vi "Extract Project Strings.vi"(8 "error in (no error)":errorcluster, 11 "New Project Wizard in":refnum<class "New Project Wizard.lvclass">) -> (0 "error out":errorcluster, 3 "New Project Wizard out":refnum<class "New Project Wizard.lvclass">)   [LabVIEW 2013, in "SET Project Editor.lvlib" / "New Project Wizard.lvclass"]
uses:
  New Project Wizard.lvclass
  New Project Wizard.lvclass/New Project Wizard.ctl
  SET Project Data/Resource Data Class/Resource Data.lvclass
  SET Project Data/Project Data Class/Project Data.lvclass
  SET Project Data/VI Class/VI Data.lvclass
  SET Project Data/Menu Class/Menu Data.lvclass
  lib/printf/messages/General/LV_Printf Msg.lvclass
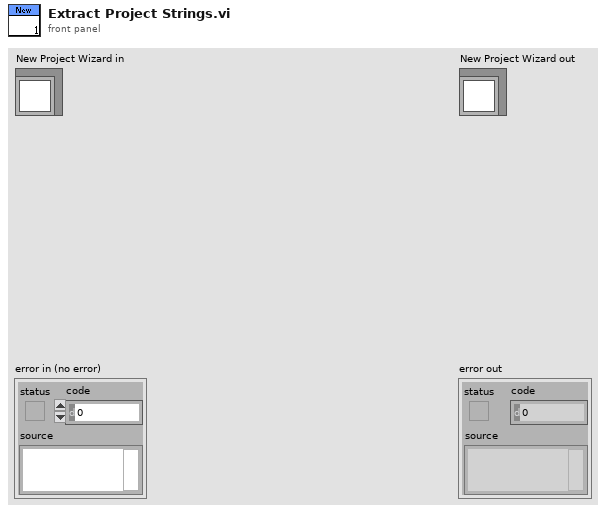
[diagram p1: front panel]
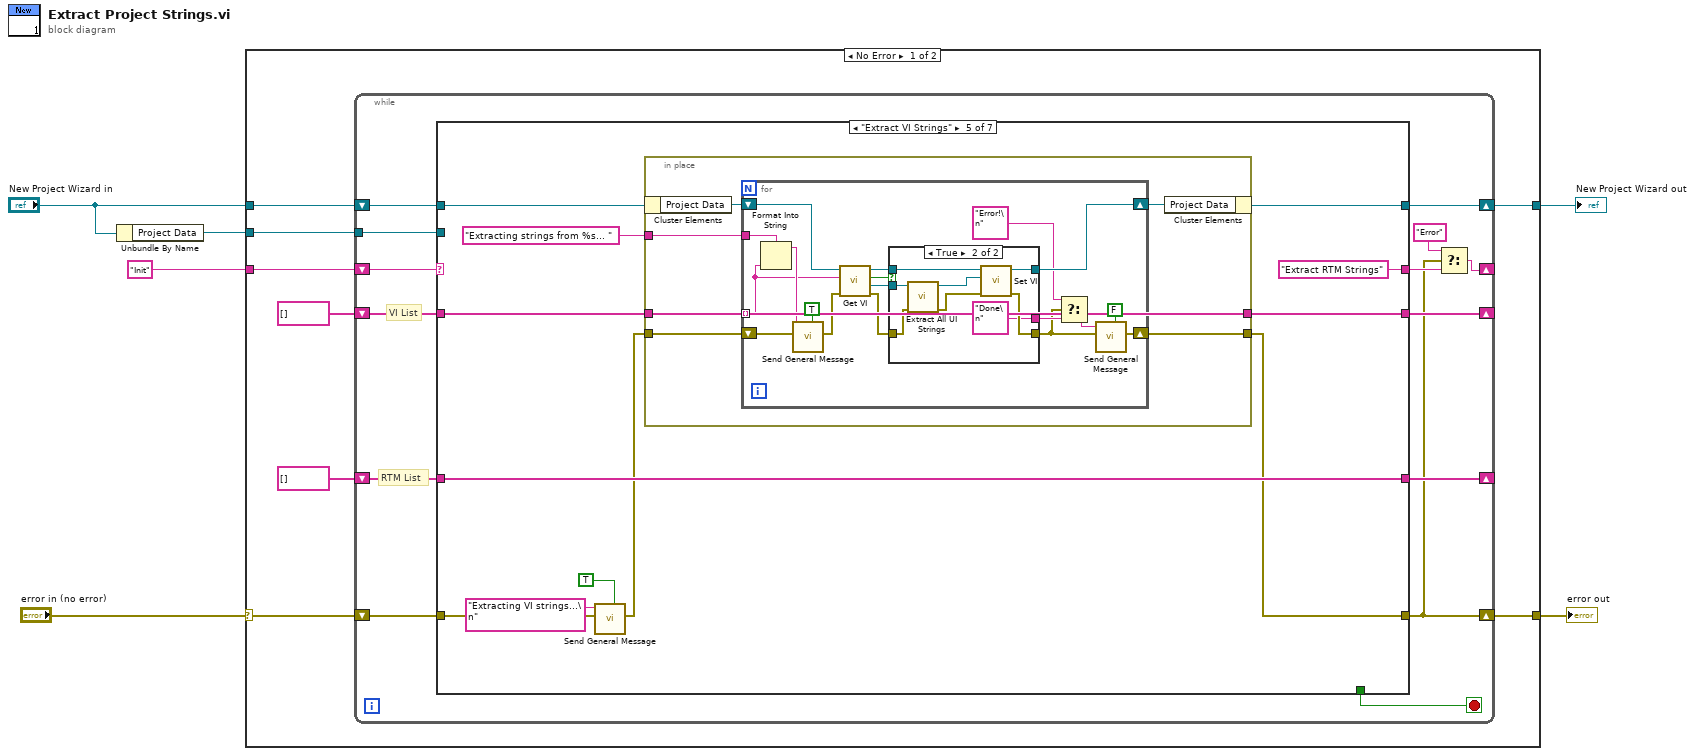
[diagram p0: block diagram]
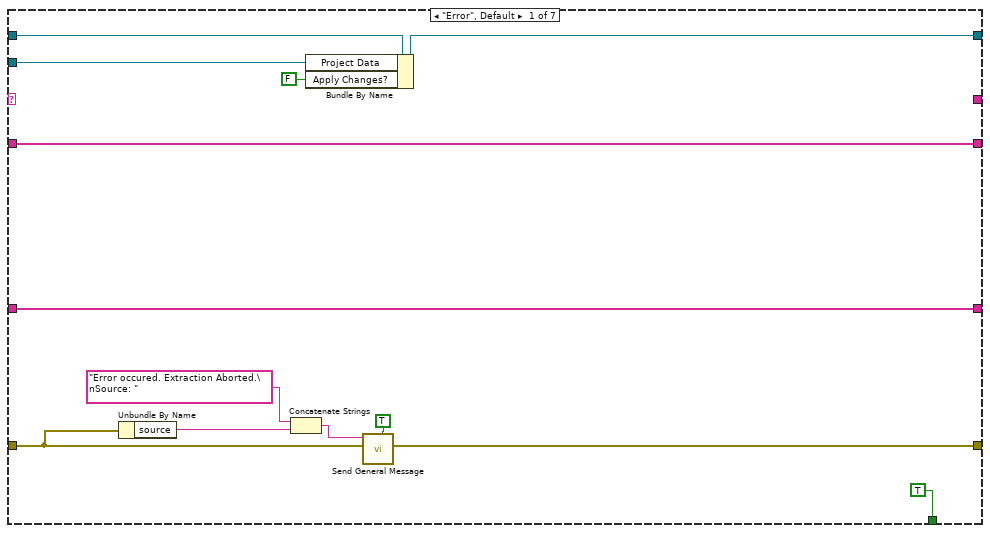
[diagram p2: hidden frame]
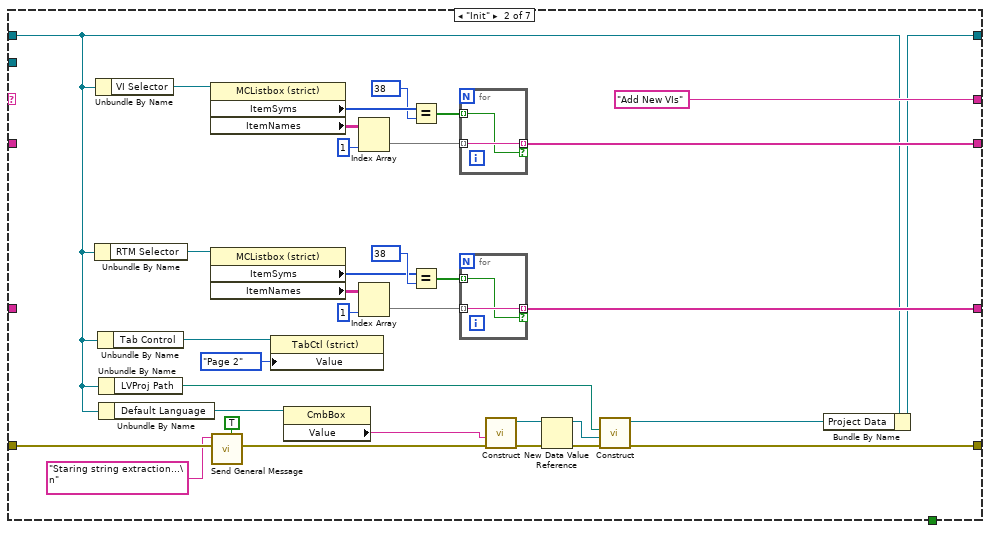
[diagram p3: hidden frame]
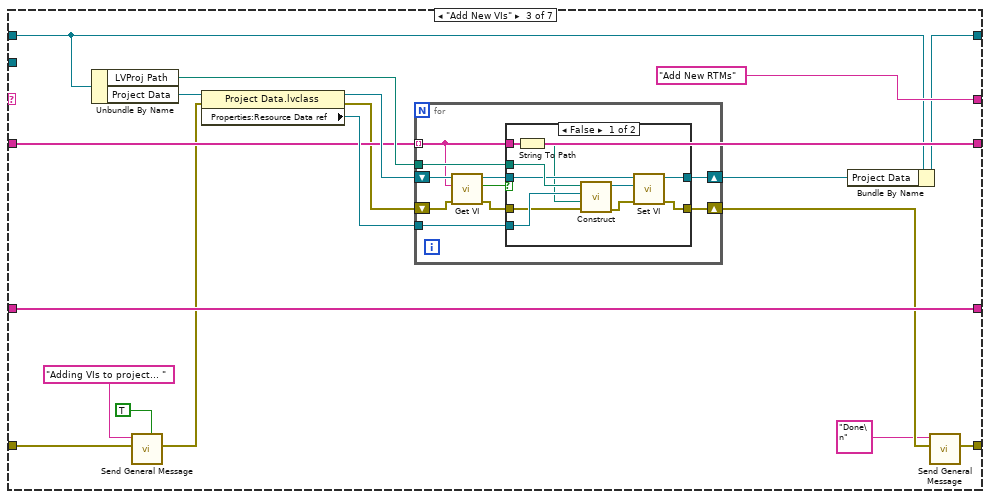
[diagram p4: hidden frame]
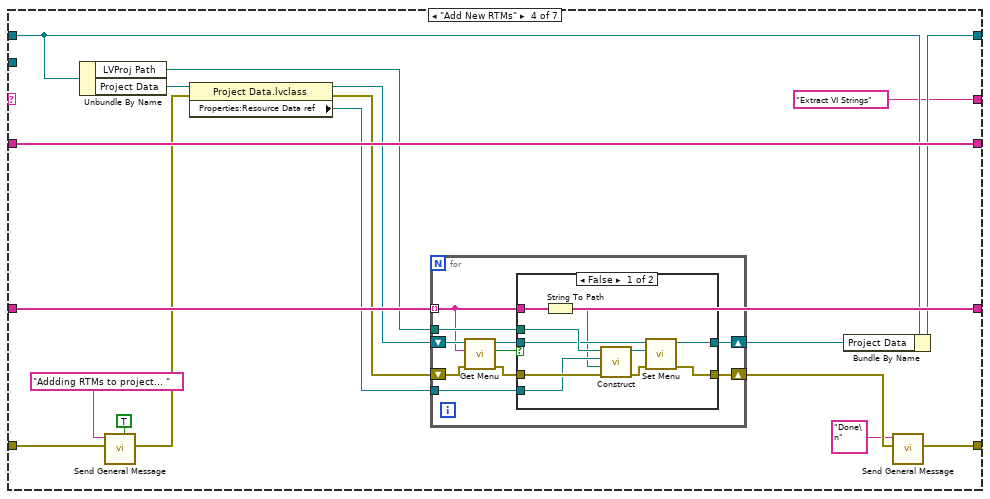
[diagram p6: hidden frame]
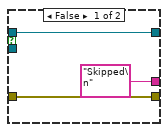
[diagram p8: hidden frame]
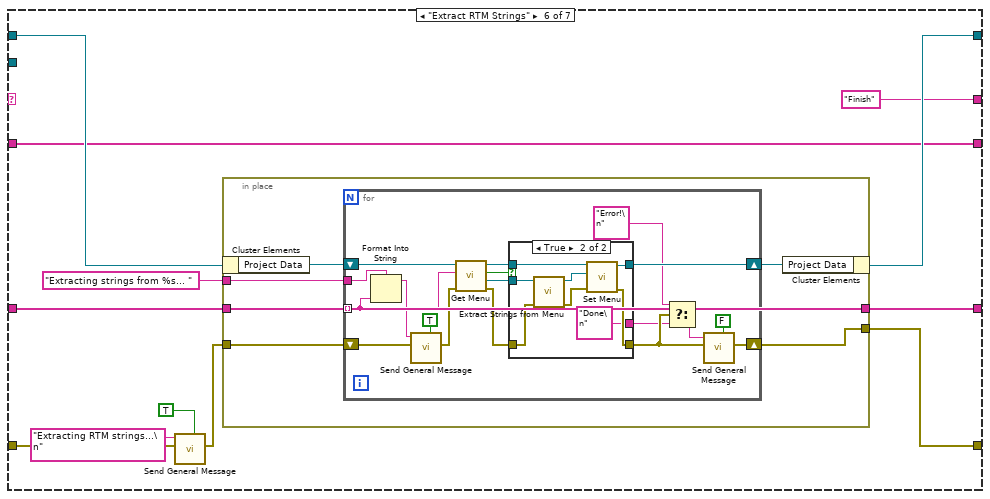
[diagram p9: hidden frame]
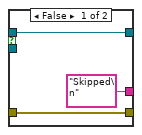
[diagram p10: hidden frame]
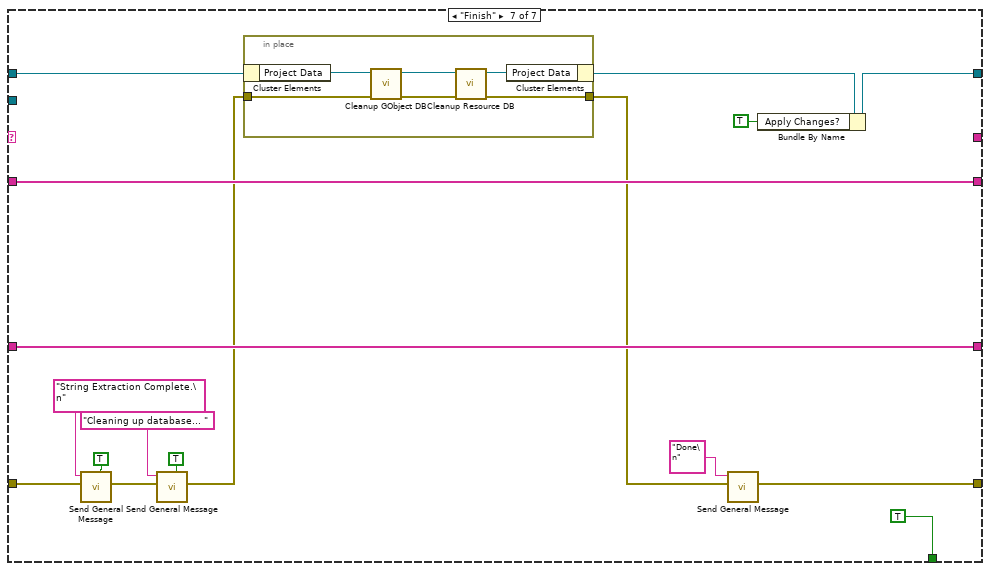
[diagram p11: hidden frame]
diagram:
  n1 = Unbundle By Name("New Project Wizard in") -> ("Project Data"=w1:refnum<class "Project Data.lvclass">)
  n2 = case shown="No Error" "error in (no error)" {
    selector: "error in (no error)" -> [w9 w278]
    tunnel: [w8 w278] -> w4
    tunnel: [w10 w277] -> w3
    tunnel: "New Project Wizard in" -> [w14 w277]
    tunnel: "Init" -> [w13 _]
    tunnel: w1 -> [w7 _]
    frame No Error {
      n3 = while {
        shift-right: [w17] -> _
        shift-left: w13 -> [w28]
        shift-right: [w22] -> w10
        shift-left: w14 -> [w27]
        shift-right: [w26] -> _
        shift-left: string[] [] -> [w25]
        shift-right: [w24] -> _
        shift-left: string[] [] -> [w23]
        shift-right: [w18] -> w8
        shift-left: w9 -> [w20]
        tunnel: w7 -> [w15]
        stop <- w21 stop-if-true
        # "RTM List"
        # "VI List"
        n4 = case shown="\"Extract VI Strings\"" w28 {
          tunnel: w27 -> [w32 w46 w90 w130 w171 w218 w267]
          tunnel: [w41 w68 w92 w135 w169 w213 w270] -> w26
          tunnel: w25 -> [w41 _ w92 w135 w170 w213 w270]
          tunnel: [w40 w60 w93 w136 w166 w214 w269] -> w24
          tunnel: w23 -> [w40 _ w93 w136 w166 w215 w269]
          tunnel: [w31 w45 w89 w129 w168 w217 w255] -> w22
          tunnel: [_ "Add New VIs" "Add New RTMs" "Extract VI Strings" "Extract RTM Strings" "Finish" _] -> w19
          tunnel: [TRUE _ _ _ _ _ TRUE] -> w21
          tunnel: w20 -> [w36 w56 w86 w126 w164 w209 w266]
          tunnel: [w37 w43 w82 w122 w165 w212 w258] -> w18
          tunnel: w15 -> [w30 _ _ _ _ _ _]
          frame "Error", Default {
            n5 = Unbundle By Name(w36) -> ("source"=w34:string)
            n6 = Concatenate Strings("Error occured. Extraction Aborted.\nSource: ", w34) -> (w33:string)
            n7 = Bundle By Name(cluster=w32, "Project Data"=w30, "Apply Changes?"=FALSE) -> (w31:refnum<class "New Project Wizard.lvclass">)
            n8 = call "Send General Message.vi"("Timestamp in message? (F)"=TRUE, "error in (no error)"=w36, "Message"=w33) -> ("error out"=w37:errorcluster)  [unwired: 8 in]
          }
          frame "Init" {
            n9 = Unbundle By Name(w46) -> ("RTM Selector"=w61:refnum<vi>)
            n10 = Unbundle By Name(w46) -> ("VI Selector"=w71:refnum<vi>)
            n11 = Unbundle By Name(w46) -> ("Tab Control"=w58:refnum<vi>)
            n12 = Unbundle By Name(w46) -> ("LVProj Path"=w47:path)
            n13 = Unbundle By Name(w46) -> ("Default Language"=w54:refnum<vi>)
            n14 = property class="MCListbox (strict)"(reference=w71) -> ("ItemSyms"=w73:i32[], "ItemNames"=w74:string[][])  [unwired: 1 in, 2 out]
            n15 = property class="MCListbox (strict)"(reference=w61) -> ("ItemSyms"=w64:i32[], "ItemNames"=w63:string[][])  [unwired: 1 in, 2 out]
            n16 = call "Send General Message.vi"("Timestamp in message? (F)"=TRUE, "error in (no error)"=w56, "Message"="Staring string extraction...\n" ("Status")) -> ("error out"=w49:errorcluster)  [unwired: 8 in]
            n17 = property class="TabCtl (strict)"(reference=w58, "Value"=enum32{"Page 1", "Page 2"}."Page 2") -> ()  [unwired: 1 in, 2 out]
            n18 = property class="CmbBox"(reference=w54) -> ("Value"=w48:string)  [unwired: 1 in, 2 out]
            n19 = Index Array(array=w74, index (col)=1 ("disabled index (col)")) -> (element=w70:string[])  [unwired: 1 in]
            n20 = Index Array(array=w63, index (col)=1 ("disabled index (col)")) -> (element=w66:string[])  [unwired: 1 in]
            n21 = Equal?(x=w73, y=38) -> (x = y?=w69:bool[])
            n22 = Equal?(x=w64, y=38) -> (x = y?=w67:bool[])
            n23 = for {
              tunnel: w70 -> [w79] mode=indexing
              tunnel: w69 -> [w78] mode=indexing
              tunnel: [w79] -> w68 mode=indexing if=w78
            }
            n24 = for {
              tunnel: w66 -> [w77] mode=indexing
              tunnel: w67 -> [w76] mode=indexing
              tunnel: [w77] -> w60 mode=indexing if=w76
            }
            n25 = call "Construct.vi"("error in (no error)"=w49, "Default Language"=w48) -> ("error out"=w51:errorcluster, "LangFile out"=w52:refnum<class "Resource Data.lvclass">)  [unwired: 8 in]
            n26 = New Data Value Reference(data value=w52, error in=w51) -> (data value reference=w53:refnum<data-value>, error out=w50:errorcluster)
            n27 = call "Construct.vi"("error in (no error)"=w50, "Resource Data ref"=w53, "Project Path"=w47) -> ("error out"=w43:errorcluster, "Project Data out"=w44:refnum<class "Project Data.lvclass">)  [unwired: 7 in]
            n28 = Bundle By Name(cluster=w46, "Project Data"=w44) -> (w45:refnum<class "New Project Wizard.lvclass">)
          }
          frame "Add New VIs" {
            n29 = Unbundle By Name(w90) -> ("LVProj Path"=w96:path, "Project Data"=w97:refnum<class "Project Data.lvclass">)
            n30 = call "Send General Message.vi"("Timestamp in message? (F)"=TRUE ("Timestamp in message? (T)"), "error in (no error)"=w86, "Message"="Adding VIs to project... ") -> ("error out"=w85:errorcluster)  [unwired: 8 in]
            n31 = property class="Project Data.lvclass"(reference=w97, error in=w85) -> (reference out=w95:refnum<class "Project Data.lvclass">, error out=w87:errorcluster, "Properties:Resource Data ref"=w94:refnum<data-value>)
            n32 = for {
              shift-right: [w106] -> w88
              shift-left: w95 -> [w107]
              shift-right: [w105] -> w83
              shift-left: w87 -> [w103]
              tunnel: w94 -> [w104]
              tunnel: w96 -> [w102]
              tunnel: w92 -> [w101] mode=indexing
              n33 = call-dynamic "Get VI.vi"("error in (no error)"=w103, "VI Path (Relative)"=w101, "ProjectData in"=w107) -> ("error out"=w99:errorcluster, "found"=w98:bool, "ProjectData out"=w100:refnum<class "Project Data.lvclass">)  [unwired: 5 in, 1 out]
              n34 = case shown="False" w98 {
                tunnel: [w117 w119] -> w106
                tunnel: [w116 w118] -> w105
                tunnel: w104 -> [w113 _]
                tunnel: w102 -> [w112 _]
                tunnel: w100 -> [w111 w119]
                tunnel: w101 -> [w110 _]
                tunnel: w99 -> [w108 w118]
                frame False {
                  n35 = String To Path(string=w110) -> (path=w109:path)
                  n36 = call "Construct.vi"("error in (no error)"=w108, "VI Path (Relative)"=w109, "Resource Data ref"=w113, "LVProject File Path (Absolute)"=w112) -> ("error out"=w115:errorcluster, "VI Data out"=w114:refnum<class "VI Data.lvclass">)  [unwired: 6 in]
                  n37 = call-dynamic "Set VI.vi"("error in (no error)"=w115, "VI Data in"=w114, "ProjectData in"=w111) -> ("error out"=w116:errorcluster, "ProjectData out"=w117:refnum<class "Project Data.lvclass">)  [unwired: 6 in, 1 out]
                }
                frame True {
                }
              }
            }
            n38 = Bundle By Name(cluster=w90, "Project Data"=w88) -> (w89:refnum<class "New Project Wizard.lvclass">)
            n39 = call "Send General Message.vi"("error in (no error)"=w83, "Message"="Done\n") -> ("error out"=w82:errorcluster)  [unwired: 9 in]
          }
          frame "Add New RTMs" {
            n40 = Unbundle By Name(w130) -> ("LVProj Path"=w134:path, "Project Data"=w137:refnum<class "Project Data.lvclass">)
            n41 = call "Send General Message.vi"("Timestamp in message? (F)"=TRUE, "error in (no error)"=w126, "Message"="Addding RTMs to project... ") -> ("error out"=w125:errorcluster)  [unwired: 8 in]
            n42 = property class="Project Data.lvclass"(reference=w137, error in=w125) -> (reference out=w133:refnum<class "Project Data.lvclass">, error out=w131:errorcluster, "Properties:Resource Data ref"=w132:refnum<data-value>)
            n43 = for {
              shift-right: [w146] -> w128
              shift-left: w133 -> [w147]
              shift-right: [w145] -> w121
              shift-left: w131 -> [w143]
              tunnel: w132 -> [w144]
              tunnel: w134 -> [w142]
              tunnel: w136 -> [w141] mode=indexing
              n44 = call-dynamic "Get Menu.vi"("error in (no error)"=w143, "Menu Path (Relative)"=w141, "ProjectData in"=w147) -> ("error out"=w138:errorcluster, "found"=w139:bool, "ProjectData out"=w140:refnum<class "Project Data.lvclass">)  [unwired: 5 in, 1 out]
              n45 = case shown="False" w139 {
                tunnel: w138 -> [w157 w158]
                tunnel: w144 -> [w156 _]
                tunnel: w142 -> [w155 _]
                tunnel: w140 -> [w154 w159]
                tunnel: [w153 w159] -> w146
                tunnel: [w151 w158] -> w145
                tunnel: w141 -> [w149 _]
                frame False {
                  n46 = String To Path(string=w149) -> (path=w148:path)
                  n47 = call "Construct.vi"("error in (no error)"=w157, "Menu Path (Relative)"=w148, "Resource Data ref"=w156, "LVProject File Path"=w155) -> ("error out"=w150:errorcluster, "Menu Data out"=w152:refnum<class "Menu Data.lvclass">)  [unwired: 6 in]
                  n48 = call-dynamic "Set Menu.vi"("error in (no error)"=w150, "RTM Data in"=w152, "ProjectData in"=w154) -> ("error out"=w151:errorcluster, "ProjectData out"=w153:refnum<class "Project Data.lvclass">)  [unwired: 6 in, 1 out]
                }
                frame True {
                }
              }
            }
            n49 = Bundle By Name(cluster=w130, "Project Data"=w128) -> (w129:refnum<class "New Project Wizard.lvclass">)
            n50 = call "Send General Message.vi"("error in (no error)"=w121, "Message"="Done\n") -> ("error out"=w122:errorcluster)  [unwired: 9 in]
          }
          frame "Extract VI Strings" {
            n51 = call "Send General Message.vi"("Timestamp in message? (F)"=TRUE, "error in (no error)"=w164, "Message"="Extracting VI strings...\n") -> ("error out"=w163:errorcluster)  [unwired: 8 in]
            n52 = in-place {
              in-place-border: w170 -> [w175]
              in-place-border: [w175] -> w169
              in-place-border: w163 -> [w174]
              in-place-border: [w173] -> w165
              in-place-border: "Extracting strings from %s... " -> [w172]
              n53 = in-place-cluster #1(w171) -> ("Project Data"=w177:refnum<class "Project Data.lvclass">)
              n54 = for {
                tunnel: w175 -> [w178] mode=indexing
                shift-right: [w189] -> w173
                shift-left: w174 -> [w183]
                shift-right: [w190] -> w176
                shift-left: w177 -> [w195]
                tunnel: w172 -> [w180]
                n55 = Format Into String(format string=w180, w178) -> (resulting string=w179:string)  [unwired: 2 in, 1 out]
                n56 = call "Send General Message.vi"("Timestamp in message? (F)"=TRUE, "error in (no error)"=w183, "Message"=w179) -> ("error out"=w182:errorcluster)  [unwired: 8 in]
                n57 = call-dynamic "Get VI.vi"("error in (no error)"=w182, "VI Path (Relative)"=w178, "ProjectData in"=w195) -> ("error out"=w193:errorcluster, "VI Data out"=w194:refnum<class "VI Data.lvclass">, "found"=w191:bool, "ProjectData out"=w192:refnum<class "Project Data.lvclass">)  [unwired: 5 in]
                n58 = case shown="True" w191 {
                  tunnel: w194 -> [_ w206]
                  tunnel: w193 -> [w198 w205]
                  tunnel: w192 -> [w197 w204]
                  tunnel: [w198 w201] -> w184
                  tunnel: [w197 w200] -> w190
                  tunnel: ["Skipped\n" "Done\n"] -> w186
                  frame False {
                  }
                  frame True {
                    n59 = call "Extract All UI Strings.vi"("error in (no error)"=w205, "LanguageData in"=w206) -> ("error out"=w202:errorcluster, "LanguageData out"=w203:refnum<class "VI Data.lvclass">)  [unwired: 8 in]
                    n60 = call-dynamic "Set VI.vi"("error in (no error)"=w202, "VI Data in"=w203, "ProjectData in"=w204) -> ("error out"=w201:errorcluster, "ProjectData out"=w200:refnum<class "Project Data.lvclass">)  [unwired: 6 in, 1 out]
                  }
                }
                n61 = Select(t="Error!\n", s=w184, f=w186) -> (s? t:f=w185:string)
                n62 = call "Send General Message.vi"("Timestamp in message? (F)"=FALSE, "error in (no error)"=w184, "Message"=w185) -> ("error out"=w189:errorcluster)  [unwired: 8 in]
              }
              n63 = in-place-cluster #1("Project Data"=w176) -> (w168:refnum<class "New Project Wizard.lvclass">)
            }
          }
          frame "Extract RTM Strings" {
            n64 = call "Send General Message.vi"("Timestamp in message? (F)"=TRUE, "error in (no error)"=w209, "Message"="Extracting RTM strings...\n") -> ("error out"=w208:errorcluster)  [unwired: 8 in]
            n65 = in-place {
              in-place-border: w215 -> [w222]
              in-place-border: [w222] -> w214
              in-place-border: w208 -> [w221]
              in-place-border: [w220] -> w212
              in-place-border: "Extracting strings from %s... " -> [w219]
              n66 = in-place-cluster #2(w218) -> ("Project Data"=w224:refnum<class "Project Data.lvclass">)
              n67 = for {
                tunnel: w222 -> [w236] mode=indexing
                shift-right: [w228] -> w220
                shift-left: w221 -> [w234]
                shift-right: [w242] -> w223
                shift-left: w224 -> [w241]
                tunnel: w219 -> [w225]
                n68 = Format Into String(format string=w225, w236) -> (resulting string=w232:string)  [unwired: 2 in, 1 out]
                n69 = call "Send General Message.vi"("Timestamp in message? (F)"=TRUE, "error in (no error)"=w234, "Message"=w232) -> ("error out"=w233:errorcluster)  [unwired: 8 in]
                n70 = call-dynamic "Get Menu.vi"("error in (no error)"=w233, "Menu Path (Relative)"=w236, "ProjectData in"=w241) -> ("error out"=w240:errorcluster, "Menu Data out"=w239:refnum<class "Menu Data.lvclass">, "found"=w238:bool, "ProjectData out"=w237:refnum<class "Project Data.lvclass">)  [unwired: 5 in]
                n71 = case shown="True" w238 {
                  tunnel: w239 -> [_ w253]
                  tunnel: w240 -> [w245 w247]
                  tunnel: w237 -> [w244 w252]
                  tunnel: [w245 w250] -> w229
                  tunnel: [w244 w251] -> w242
                  tunnel: ["Skipped\n" "Done\n"] -> w226
                  frame False {
                  }
                  frame True {
                    n72 = call "Extract Strings from Menu.vi"("error in (no error)"=w247, "Object in"=w253) -> ("error out"=w249:errorcluster, "Object out"=w248:refnum<class "Menu Data.lvclass">)  [unwired: 8 in]
                    n73 = call-dynamic "Set Menu.vi"("error in (no error)"=w249, "RTM Data in"=w248, "ProjectData in"=w252) -> ("error out"=w250:errorcluster, "ProjectData out"=w251:refnum<class "Project Data.lvclass">)  [unwired: 6 in, 1 out]
                  }
                }
                n74 = Select(t="Error!\n", s=w229, f=w226) -> (s? t:f=w230:string)
                n75 = call "Send General Message.vi"("Timestamp in message? (F)"=FALSE, "error in (no error)"=w229, "Message"=w230) -> ("error out"=w228:errorcluster)  [unwired: 8 in]
              }
              n76 = in-place-cluster #2("Project Data"=w223) -> (w217:refnum<class "New Project Wizard.lvclass">)
            }
          }
          frame "Finish" {
            n77 = call "Send General Message.vi"("Timestamp in message? (F)"=TRUE, "error in (no error)"=w266, "Message"="String Extraction Complete.\n") -> ("error out"=w261:errorcluster)  [unwired: 8 in]
            n78 = call "Send General Message.vi"("Timestamp in message? (F)"=TRUE, "error in (no error)"=w261, "Message"="Cleaning up database... ") -> ("error out"=w260:errorcluster)  [unwired: 8 in]
            n79 = in-place {
              in-place-border: w260 -> [w272]
              in-place-border: [w271] -> w259
              n80 = in-place-cluster #3(w267) -> ("Project Data"=w274:refnum<class "Project Data.lvclass">)
              n81 = call "Cleanup GObject DB.vi"("error in (no error)"=w272, "Project Data in"=w274) -> ("error out"=w275:errorcluster, "Project Data out"=w276:refnum<class "Project Data.lvclass">)  [unwired: 8 in]
              n82 = call-dynamic "Cleanup Resource DB.vi"("error in (no error)"=w275, "ProjectData in"=w276) -> ("error out"=w271:errorcluster, "ProjectData out"=w273:refnum<class "Project Data.lvclass">)  [unwired: 8 in]
              n83 = in-place-cluster #3("Project Data"=w273) -> (w256:refnum<class "New Project Wizard.lvclass">)
            }
            n84 = call "Send General Message.vi"("error in (no error)"=w259, "Message"="Done\n") -> ("error out"=w258:errorcluster)  [unwired: 9 in]
            n85 = Bundle By Name(cluster=w256, "Apply Changes?"=TRUE) -> (w255:refnum<class "New Project Wizard.lvclass">)
          }
        }
        n86 = Select(t="Error", s=w18, f=w19) -> (s? t:f=w17:string)
      }
    }
    frame Error {
    }
  }
  "error out" <- w4
  "New Project Wizard out" <- w3
